vi "Refresh Device Info.vi"(8 "error in (no error)":errorcluster, 11 "Device in":refnum<class "Device.lvclass">) -> (0 "error out":errorcluster, 3 "Device out":refnum<class "Device.lvclass">)   [LabVIEW 2020, in "PicoG-App.lvlib" / "Device.lvclass"]
uses:
  Device.lvclass
  Builds/picoG/ppl/PicoG-Core.lvlibp/PicoG-Processor/PicoG-Core/DeployResource/DeployResource.lvclass
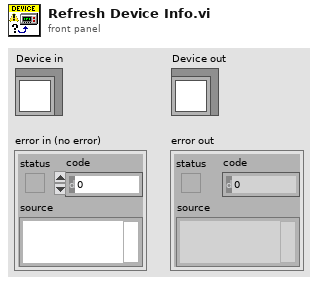
[diagram p1: front panel]
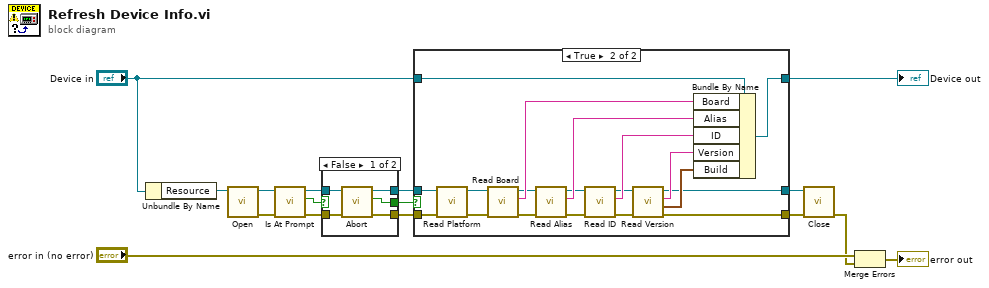
[diagram p0: block diagram]
diagram:
  n1 = Unbundle By Name("Device in") -> ("Resource"=w7:refnum<class "DeployResource.lvclass">)
  n2 = call-dynamic "Open.vi"("DeployResource in"=w7) -> ("error out"=w5:errorcluster, "DeployResource out"=w6:refnum<class "DeployResource.lvclass">)  [unwired: 9 in]
  n3 = call-dynamic "Is At Prompt.vi"("error in (no error)"=w5, "DeployResource in"=w6) -> ("error out"=w14:errorcluster, "At Prompt?"=w15:bool, "DeployResource out"=w13:refnum<class "DeployResource.lvclass">)  [unwired: 6 in, 1 out]
  n4 = case shown="False" w15 {
    selector: w15 -> [_ w24]
    tunnel: w14 -> [w20 w22]
    tunnel: w13 -> [w21 w23]
    tunnel: [w19 w24] -> w10
    tunnel: [w18 w23] -> w11
    tunnel: [w17 w22] -> w9
    frame False {
      n5 = call-dynamic "Abort.vi"("error in (no error)"=w20, "DeployResource in"=w21) -> ("error out"=w17:errorcluster, "Stopped?"=w19:bool, "DeployResource out"=w18:refnum<class "DeployResource.lvclass">)  [unwired: 6 in, 1 out]
    }
    frame True {
    }
  }
  n6 = case shown="True" w10 {
    tunnel: "Device in" -> [w25 w46]
    tunnel: w11 -> [w27 w44]
    tunnel: w9 -> [w26 w43]
    tunnel: [w25 w45] -> w8
    tunnel: [w27 w30] -> w4
    tunnel: [w26 w28] -> w3
    frame False {
      # "#ERROR"
    }
    frame True {
      n7 = call "Read Platform.vi"("error in (no error)"=w43, "DeployResource in"=w44) -> ("error out"=w41:errorcluster, "DeployResource out"=w42:refnum<class "DeployResource.lvclass">)  [unwired: 7 in, 1 out]
      n8 = call "Read Board.vi"("error in (no error)"=w41, "DeployResource in"=w42) -> ("error out"=w38:errorcluster, "Board"=w40:string, "DeployResource out"=w39:refnum<class "DeployResource.lvclass">)  [unwired: 7 in]
      n9 = call "Read Alias.vi"("error in (no error)"=w38, "DeployResource in"=w39) -> ("error out"=w35:errorcluster, "Alias"=w37:string, "DeployResource out"=w36:refnum<class "DeployResource.lvclass">)  [unwired: 7 in]
      n10 = call "Read ID.vi"("error in (no error)"=w35, "DeployResource in"=w36) -> ("error out"=w29:errorcluster, "ID"=w34:string, "DeployResource out"=w33:refnum<class "DeployResource.lvclass">)  [unwired: 7 in]
      n11 = call "Read Version.vi"("error in (no error)"=w29, "DeployResource in"=w33) -> ("error out"=w28:errorcluster, "Build"=w31:timestamp, "Version"=w32:string, "DeployResource out"=w30:refnum<class "DeployResource.lvclass">)  [unwired: 6 in]
      n12 = Bundle By Name(cluster=w46, "Board"=w40, "Alias"=w37, "ID"=w34, "Version"=w32, "Build"=w31) -> (w45:refnum<class "Device.lvclass">)
    }
  }
  "Device out" <- w8
  n13 = call-dynamic "Close.vi"("error in (no error)"=w3, "DeployResource in"=w4) -> ("error out"=w1:errorcluster)  [unwired: 8 in, 1 out]
  n14 = Merge Errors("error in (no error)", w1) -> (→"error out":errorcluster)
